vi "Delete BuildSpec Tags.vi"(8 "error in (no error)":errorcluster, 10 "Tag Names":string[](array[string]), 11 "ProjectItem in":refnum<vi>) -> (0 "error out":errorcluster, 2 "Deleted ?":bool[](array[boolean]), 3 "ProjectItem out":refnum<vi>)   [LabVIEW 2019, in "Project Sync Tools.lvclass"]
uses:
  Project Sync Tools.lvclass
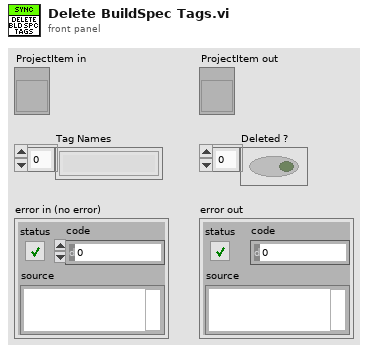
[diagram p1: front panel]
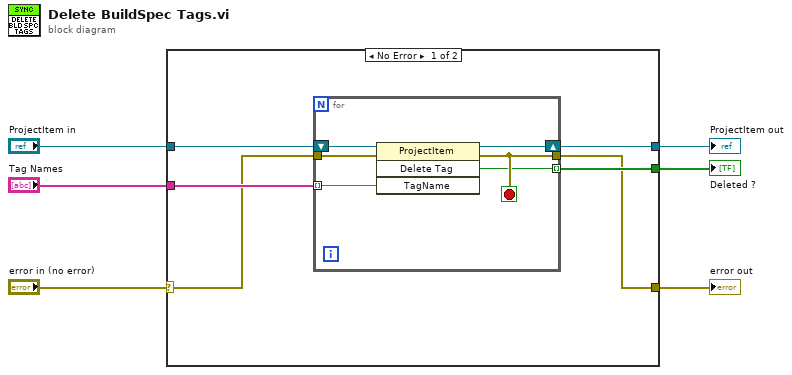
[diagram p0: block diagram]
diagram:
  n1 = case shown="No Error" "error in (no error)" {
    selector: "error in (no error)" -> [w7 w20]
    tunnel: [w12 _] -> w6
    tunnel: [w11 w19] -> w5
    tunnel: [w10 w20] -> w4
    tunnel: "Tag Names" -> [w9 _]
    tunnel: "ProjectItem in" -> [w8 w19]
    frame No Error {
      n2 = for {
        tunnel: w9 -> [w17] mode=indexing
        tunnel: w7 -> [w16]
        shift-right: [w15] -> w11
        shift-left: w8 -> [w18]
        tunnel: [w14] -> w10
        tunnel: [w13] -> w12 mode=indexing
        stop <- w14 stop-if-true
        n3 = invoke class="ProjectItem" method="Delete Tag"(reference=w18, error in=w16, "TagName"=w17) -> (reference out=w15:refnum<vi>, error out=w14:errorcluster, "DeleteTag"=w13:bool)  [unwired: 1 in, 1 out]
      }
    }
    frame Error {
    }
  }
  "Deleted ?" <- w6
  "ProjectItem out" <- w5
  "error out" <- w4
